vi "未命名 3.vi"() -> ()   [LabVIEW 2010]
uses:
  <vilib>/addons/Modulation/Analog/controls/Complex Data Waveform.ctl
  <vilib>/addons/Modulation/Digital/General/MT Generate Bits (Galois, PN Order).vi
  <vilib>/addons/Modulation/Digital/Impairments/Fading Profiles/MT Rician Fading Profile (Jakes).vi
  <vilib>/Analysis/2dsp.llb/Complex FFT.vi
  <vilib>/imath/engines/lvmath2/RunTimeEngine/ErrorHandling/NIMS_Finalize Error.vi
  <vilib>/imath/engines/lvmath2/RunTimeEngine/Managers/WorkSpace/UID Generator.vi
  <vilib>/imath/engines/lvmath2/RunTimeEngine/Managers/SymbolTable/Clear UID.vi
  <vilib>/imath/engines/lvmath2/RunTimeEngine/NodeEndStatement/NIMS_NodeEndStatement_Output.vi
  <instcachedir>/0/NIMS_NodeEndStatement_Output_53EC0D466D134D7ABD903AC30B43404B.lvgen/NIMS_NodeEndStatement_Output_53EC0D466D134D7ABD903AC30B43404B_000.vi
  <vilib>/imath/engines/lvmath2/RunTimeEngine/BuiltInFunctions/length/NIMS_length(GV).vi
  <instcachedir>/0/NIMS_length(GV)_08A3D13377FD4E4B96F5795FBF3698FA.lvgen/NIMS_length(GV)_08A3D13377FD4E4B96F5795FBF3698FA_002.vi
  <vilib>/imath/engines/lvmath2/RunTimeEngine/RunTimeType/NIMS_RunTimeType_From StrictType (excl LVString).vi
  <vilib>/imath/engines/lvmath2/RunTimeEngine/LocalVariableDefStatement/MC_LocalVariableDefStatement_Display.vi
  <vilib>/imath/engines/lvmath2/RunTimeEngine/BuiltInFunctions/zeros/NIMS_V=zeros(I32,I32).vi
  <vilib>/imathl/engines/lvmath/Functions/Error Handling/Create Error.vi
  <vilib>/imath/engines/lvmath2/RunTimeEngine/RangeToken/NIMS_Range_R2 - Integer.vi
  <instcachedir>/0/NIMS_Range_R2 - Integer_217CA55F27D14E80B3D190635C7B3F47.lvgen/NIMS_Range_R2 - Integer_217CA55F27D14E80B3D190635C7B3F47_000.vi
  <vilib>/imath/engines/lvmath2/RunTimeEngine/CommandStatement/MC_CommandStatement_break.vi
  <vilib>/imath/engines/lvmath2/RunTimeEngine/VariableToken/Read/NIMS_Get Elements - RV(_) - Check.vi
  <instcachedir>/0/NIMS_Get Elements - RV(_) - Check_1F6F8656162345078B1D4DC9877DFAE9.lvgen/NIMS_Get Elements - RV(_) - Check_1F6F8656162345078B1D4DC9877DFAE9_004.vi
  <vilib>/imath/engines/lvmath2/RunTimeEngine/ReplaceToken/NIMS_Replace - Check Linear.vi
  <instcachedir>/0/NIMS_Replace - Check Linear_662D5651E4E34E0584DA82A256193A4C.lvgen/NIMS_Replace - Check Linear_662D5651E4E34E0584DA82A256193A4C_002.vi
  <vilib>/imath/engines/lvmath2/RunTimeEngine/ReplaceToken/NIMS_Replace - Size Check _(_)=S.vi
  <instcachedir>/0/NIMS_Replace - Size Check _(_)=S_6CAC13ACC74349C582FDAB09BCDAB70F.lvgen/NIMS_Replace - Size Check _(_)=S_6CAC13ACC74349C582FDAB09BCDAB70F_001.vi
  <vilib>/imath/engines/lvmath2/RunTimeEngine/ReplaceToken/NIMS_Replace - V(S)=S.vi
  <instcachedir>/0/NIMS_Replace - V(S)=S_78FDB6CCD265407D8926E4CF958018EB.lvgen/NIMS_Replace - V(S)=S_78FDB6CCD265407D8926E4CF958018EB_001.vi
  <vilib>/Analysis/2dsp.llb/Inverse Complex FFT.vi
  <vilib>/addons/Modulation/niDMT.lvlib
  <vilib>/Analysis/NI_AALPro.lvlib
  <vilib>/addons/Modulation/niAMT.lvlib
  <vilib>/addons/Adaptive Filters/NI_AdaptiveFilter.lvlib
  <vilib>/addons/Modulation/Digital/Impairments/MT Apply Flat Fading Profile.vi
  <vilib>/imath/engines/lvmath2/RunTimeEngine/Managers/SymbolTable/NIMS_WorkSpace.lvlib
  <vilib>/addons/Adaptive Filters/Analysis/AFT Set Coefficients (FIR, Complex).vi
  <vilib>/addons/Adaptive Filters/Create/AFT Create FIR LMS (Complex).vi
  <vilib>/imath/engines/lvmath2/RunTimeEngine/BuiltInFunctions/zeros/NIMS_M=zeros(I32,I32).vi
  <vilib>/imath/engines/lvmath2/RunTimeEngine/ReplaceToken/NIMS_Replace - M(S,S)=S.vi
  <vilib>/imath/engines/lvmath2/RunTimeEngine/ReplaceToken/NIMS_Replace - Check Row.vi
  <vilib>/imath/engines/lvmath2/RunTimeEngine/ReplaceToken/NIMS_Replace - Check Column.vi
  <vilib>/imath/engines/lvmath2/RunTimeEngine/ReplaceToken/NIMS_Replace - Size Check M(_,_)=S.vi
  <vilib>/imath/engines/lvmath2/RunTimeEngine/ErrorHandling/NIMS_Create Error From Enums.vi
  <vilib>/addons/Adaptive Filters/Processing/AFT Filter Signal (Real, PtByPt).vi
  <vilib>/measure/NI_MABase.lvlib
panel:
  out "filter_out 5":dbl[](graph)
  out "coe":cdb[](array[numeric])
  out "filter_out 4":dbl[](graph)
  out "filter_out 3":dbl[](graph)
  out "filter_out 2":dbl[](graph)
  out "波形图 5":dbl[](graph)
  out "子数组":dbl[](graph)
  out "dout":cdb[][](array[numeric])
  out "波形图 4":dbl[](graph)
  out "波形图 3":dbl[](graph)
  out "波形图 2":dbl[](graph)
  out "波形图":dbl[](graph)
  out "constellation graph 2":T1(graph) caption="constellation graph"
  out "TX Constellation 2":T2(graph) caption="TX Constellation"
  out "Y":dbl[](graph)
  out "filter_out":dbl[](graph)
  out "TX Constellation":T2(graph)
  out "constellation graph":T1(graph)
  out "X":dbl[](graph)
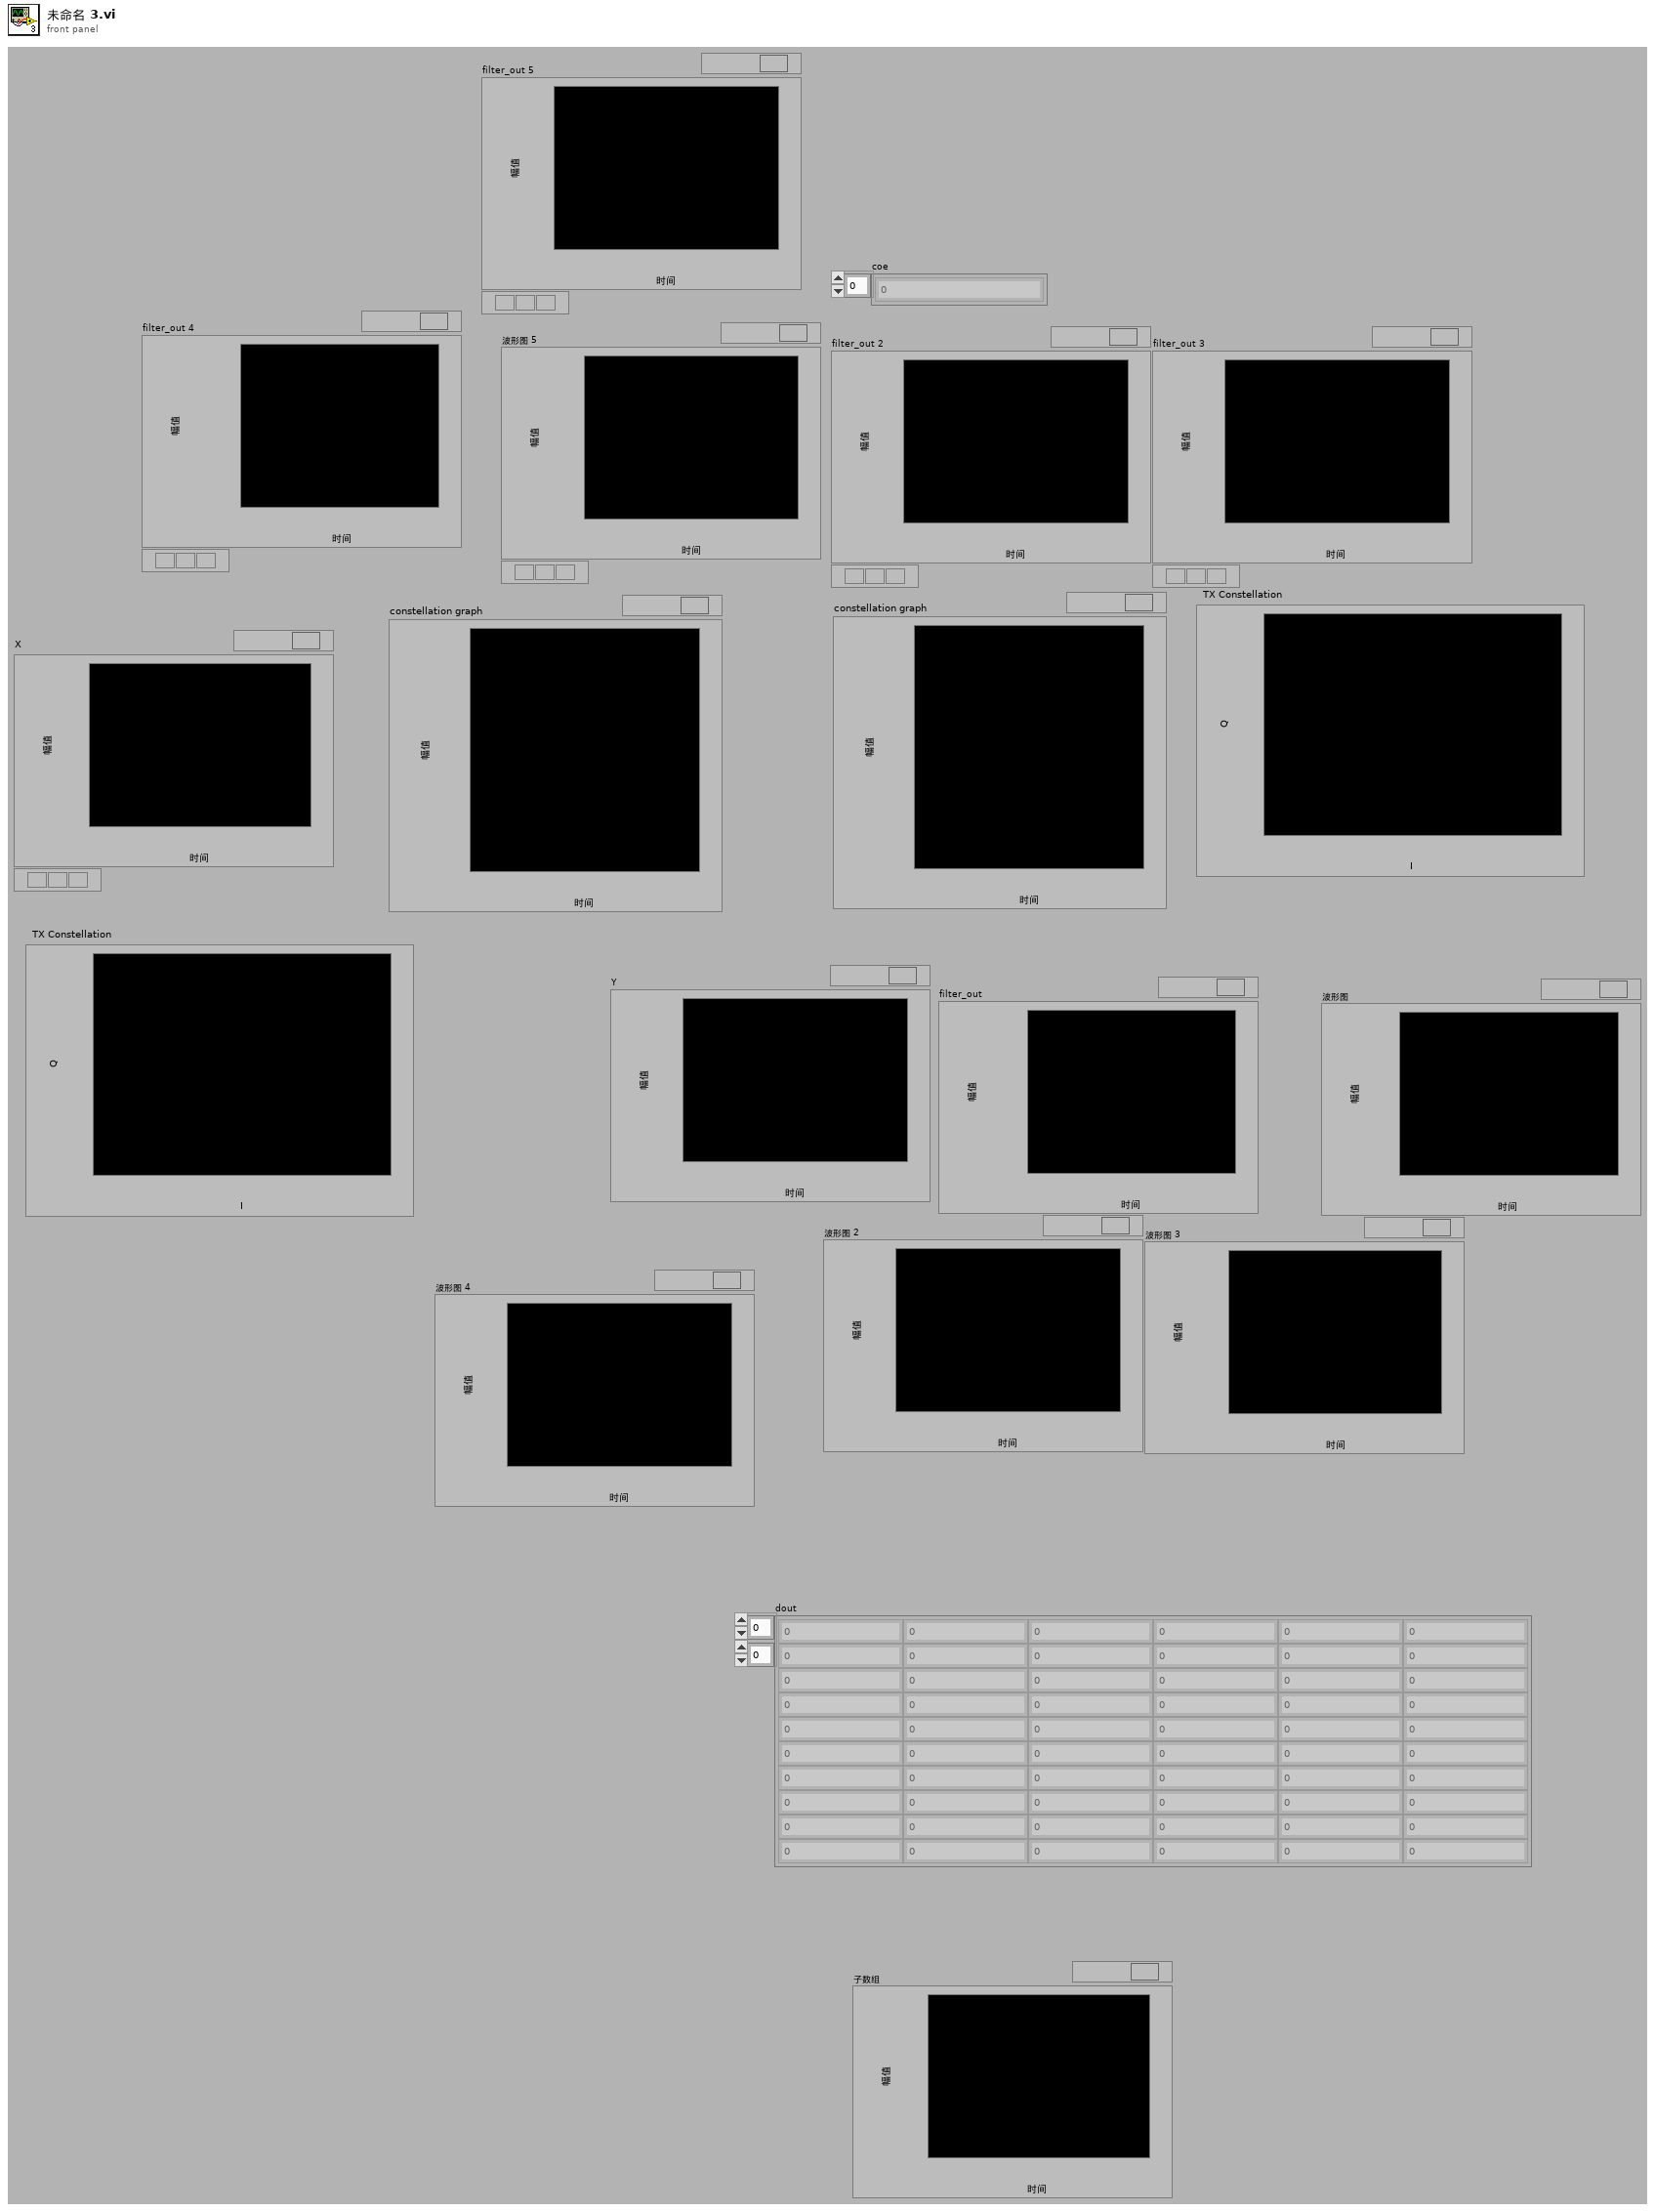
[diagram p1: front panel]
types:
  T1 = cluster{"constellation":dbl[], "oversampled data":dbl[]}[]
  T2 = cluster{"Decimated Array":dbl[], "Decimated Array":dbl[]}[]
  T3 = typedef "niAMT.lvlib/Complex Data Waveform.ctl" = cluster{"t0":dbl, "dt":dbl, "Y":cdb[]}
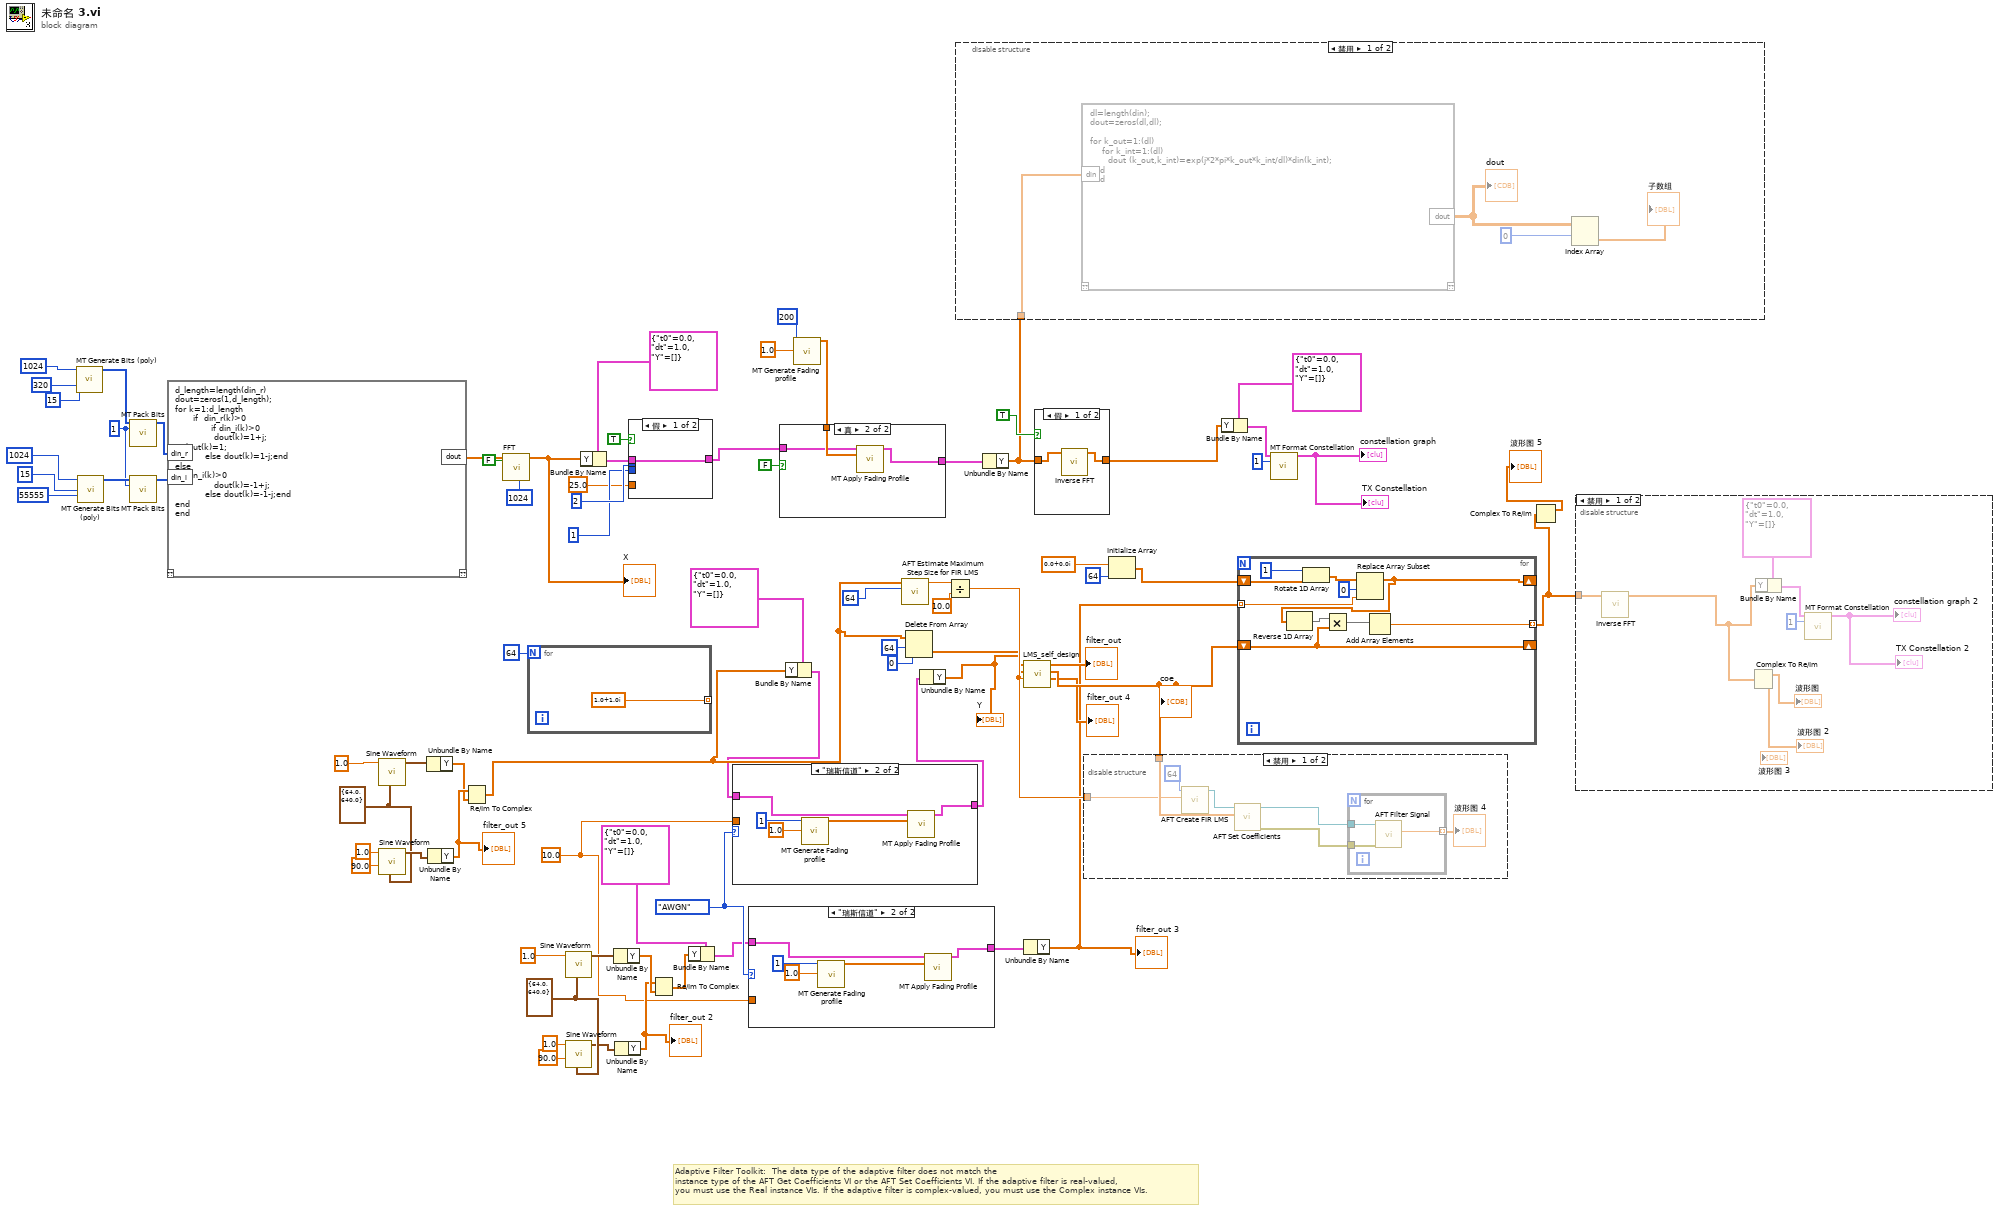
[diagram p0: block diagram]
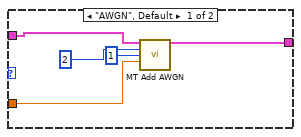
[diagram p3: hidden frame]
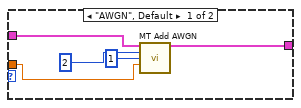
[diagram p6: hidden frame]
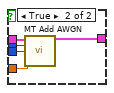
[diagram p8: hidden frame]
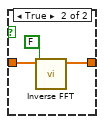
[diagram p9: hidden frame]
diagram:
  w4 = cluster{"Fs":dbl, "#s":dbl} {"Fs"=64.0, "#s"=640.0} ("sampling info")
  w23 = 10.0 ("Eb/N0 (10 dB)")
  w32 = cluster{"Fs":dbl, "#s":dbl} {"Fs"=64.0, "#s"=640.0} ("sampling info")
  w36 = enum16{"AWGN", "瑞斯信道"}."AWGN"
  w71 = 1 ("bits per integer")
  # "Adaptive Filter Toolkit:  The data type of the adaptive filter does not match the \ninstance type of the AFT Get Coefficients VI or the AFT Set Coefficients VI. If the adaptive filter is real-valued, \nyou must use the Real instance VIs. If the adaptive filter is complex-valued, you must use the Complex instance VIs."
  n1 = call-poly <vilib>:"MT Generate Bits (poly).vi"("total bits (128)"=1024, "PN sequence order (9)"=15, "seed in (0xD6BF7DF2)"=320) -> ("output bit stream"=w77:i8[])  [unwired: 10 in, 2 out]
  n2 = call-poly <vilib>:"MT Generate Bits (poly).vi"("total bits (128)"=1024, "PN sequence order (9)"=15, "seed in (0xD6BF7DF2)"=55555) -> ("output bit stream"=w73:i8[])  [unwired: 10 in, 2 out]
  n3 = call <vilib>:"MT Pack Bits.vi"("input bit stream"=w77, "bits per integer"=w71) -> ("output integers"=w68:i32[])  [unwired: 12 in, 1 out]
  n4 = call <vilib>:"MT Pack Bits.vi"("input bit stream"=w73, "bits per integer"=w71) -> ("output integers"=w69:i32[])  [unwired: 12 in, 1 out]
  n5 = mathscript code="d_length=length(din_r)\ndout=zeros(1,d_length);\nfor k=1:d_length\n      if  din_r(k)>0\n            if din_i(k)>0\n             dout(k)=1+j;\n%dout(k)=1;\n          else dout(k)=1-j;end\nelse   \n if din_i(k)>0\n             dout(k)=-1+j;\n          else dout(k)=-1-j;end\nend\nend"("din_r"=w68, "din_i"=w69) -> ("dout"=w56:cdb[])  [unwired: 1 in, 1 out]
  n6 = call <vilib>:"Sine Waveform.vi"("sampling info"=w4, "frequency"=1.0) -> ("signal out"=w8:waveform(dbl))  [unwired: 8 in, 1 out]
  n7 = call <vilib>:"Sine Waveform.vi"("sampling info"=w4, "phase"=90.0, "frequency"=1.0) -> ("signal out"=w9:waveform(dbl))  [unwired: 7 in, 1 out]
  n8 = Unbundle By Name(w8) -> ("Y"=w10:dbl[])
  n9 = Unbundle By Name(w9) -> ("Y"=w11:dbl[])
  "filter_out 5" <- w11
  n10 = Re/Im To Complex(1:w10, 2:w11) -> (0:w2:cdb[])
  n11 = call-poly <vilib>:"FFT.vi"("FFT size"=1024, "shift?"=FALSE, "X"=w56) -> ("FFT {X}"=w47:cdb[])  [unwired: 7 in, 1 out]
  "X" <- w47
  n12 = for {
    N: 64 -> [_]
    tunnel: [cdb 1.0+1.0i] -> _ mode=indexing
  }
  n13 = call <vilib>:"Sine Waveform.vi"("sampling info"=w32, "frequency"=1.0) -> ("signal out"=w31:waveform(dbl))  [unwired: 8 in, 1 out]
  n14 = call <vilib>:"Sine Waveform.vi"("sampling info"=w32, "phase"=90.0, "frequency"=1.0) -> ("signal out"=w30:waveform(dbl))  [unwired: 7 in, 1 out]
  n15 = Bundle By Name(cluster=T3 {"t0"=0.0, "dt"=1.0, "Y"=[]} ("input complex waveform"), "Y"=w47) -> (w65:T3)
  n16 = Unbundle By Name(w31) -> ("Y"=w29:dbl[])
  n17 = Unbundle By Name(w30) -> ("Y"=w25:dbl[])
  "filter_out 2" <- w25
  n18 = case shown="假" TRUE {
    tunnel: 2 ("samples per symbol (16)") -> [_ w85]
    tunnel: w65 -> [w80 w84]
    tunnel: 1 ("bits per symbol (1)") -> [_ w83]
    tunnel: 25.0 ("Eb/N0 (10 dB)") -> [_ w82]
    tunnel: [w80 w81] -> w51
    frame False {
    }
    frame True {
      n19 = call <vilib>:"MT Add AWGN.vi"("input complex waveform"=w84, "samples per symbol (16)"=w85, "bits per symbol (1)"=w83, "Eb/N0 (10 dB)"=w82) -> ("output complex waveform"=w81:T3)  [unwired: 9 in, 2 out]
    }
  }
  n20 = Re/Im To Complex(1:w29, 2:w25) -> (0:w15:cdb[])
  n21 = Bundle By Name(cluster=T3 {"t0"=0.0, "dt"=1.0, "Y"=[]} ("input complex waveform"), "Y"=w15) -> (w16:T3)
  n22 = case shown="\"瑞斯信道\"" w36 {
    tunnel: [w88 w92] -> w27
    tunnel: w16 -> [w87 w91]
    tunnel: w23 -> [w86 _]
    frame "AWGN", Default {
      n23 = call <vilib>:"MT Add AWGN.vi"("input complex waveform"=w87, "samples per symbol (16)"=2, "bits per symbol (1)"=1, "Eb/N0 (10 dB)"=w86) -> ("output complex waveform"=w88:T3)  [unwired: 9 in, 2 out]
    }
    frame "瑞斯信道" {
      n24 = call-poly <vilib>:"MT Generate Fading profile.vi"("profile length (samples)"=1, "sampling frequency (Hz)"=1.0) -> ("fading profile"=w95:cdb[])  [unwired: 11 in, 2 out]
      n25 = call-poly <vilib>:"MT Apply Fading Profile.vi"("input complex waveform"=w91, "fading profile"=w95) -> ("output complex waveform"=w92:T3)  [unwired: 12 in, 1 out]
    }
  }
  n26 = Bundle By Name(cluster=T3 {"t0"=0.0, "dt"=1.0, "Y"=[]} ("input complex waveform"), "Y"=w2) -> (w1:T3)
  n27 = case shown="\"瑞斯信道\"" w36 {
    tunnel: [w98 w101] -> w43
    tunnel: w1 -> [w97 w102]
    tunnel: w23 -> [w96 _]
    frame "AWGN", Default {
      n28 = call <vilib>:"MT Add AWGN.vi"("input complex waveform"=w97, "samples per symbol (16)"=2, "bits per symbol (1)"=1, "Eb/N0 (10 dB)"=w96) -> ("output complex waveform"=w98:T3)  [unwired: 9 in, 2 out]
    }
    frame "瑞斯信道" {
      n29 = call-poly <vilib>:"MT Generate Fading profile.vi"("profile length (samples)"=1, "sampling frequency (Hz)"=1.0) -> ("fading profile"=w105:cdb[])  [unwired: 11 in, 2 out]
      n30 = call-poly <vilib>:"MT Apply Fading Profile.vi"("input complex waveform"=w102, "fading profile"=w105) -> ("output complex waveform"=w101:T3)  [unwired: 12 in, 1 out]
    }
  }
  n31 = call-poly <vilib>:"MT Generate Fading profile.vi"("profile length (samples)"=200, "sampling frequency (Hz)"=1.0) -> ("fading profile"=w52:cdb[])  [unwired: 11 in, 2 out]
  n32 = case shown="真" FALSE {
    tunnel: w52 -> [_ w109]
    tunnel: w51 -> [w106 w108]
    tunnel: [w106 w107] -> w50
    frame False {
    }
    frame True {
      n33 = call-poly <vilib>:"MT Apply Fading Profile.vi"("input complex waveform"=w108, "fading profile"=w109) -> ("output complex waveform"=w107:T3)  [unwired: 12 in, 1 out]
    }
  }
  n34 = call <vilib>:"AFT Estimate Maximum Step Size for FIR LMS.vi"("filter length"=64, "x(n)"=w2) -> ("maximum step size"=w22:dbl)  [unwired: 8 in, 1 out]
  n35 = Delete From Array(array=w2, length=64 ("长度"), index=0 ("索引")) -> (deleted portion=w14:cdb[])  [unwired: 1 out]
  n36 = Unbundle By Name(w43) -> ("Y"=w13:cdb[])
  "Y" <- w13
  n37 = Divide(x=w22, y=10.0) -> (x/y=w17:dbl)
  n38 = Unbundle By Name(w50) -> ("Y"=w37:cdb[])
  n39 = disable-structure shown="禁用" {
    disable-tunnel: w37 -> [w110 _]
    frame Disabled {
      n40 = mathscript code="dl=length(din);\ndout=zeros(dl,dl);\n\nfor k_out=1:(dl)\n    for k_int=1:(dl)\n      dout (k_out,k_int)=exp(j*2*pi*k_out*k_int/dl)*din(k_int);\nend\nend"("din"=w110) -> ("dout"=w113:cdb[][])  [unwired: 1 in, 1 out]
      "dout" <- w113
      n41 = Index Array(array=w113, index (row)=0 ("索引 (行)")) -> (element=→"子数组":cdb[])  [unwired: 1 in]
    }
    frame Enabled {
    }
  }
  n42 = call "LMS_self_design.vi"("step_delta"=w17, "train"=w14, "sig"=w13) -> ("error"=→"filter_out 4":dbl[], "coe"=w42:cdb[], "filter_out"=→"filter_out":cdb[])  [unwired: 6 in]
  "coe" <- w42
  n43 = Unbundle By Name(w27) -> ("Y"=w3:cdb[])
  "filter_out 3" <- w3
  n44 = case shown="假" TRUE {
    tunnel: [w257 w259] -> w41
    tunnel: w37 -> [w256 w258]
    frame False {
      n45 = call-poly <vilib>:"Inverse FFT.vi"("FFT {X}"=w256) -> ("X"=w257:cdb[])  [unwired: 9 in, 1 out]
    }
    frame True {
      n46 = call-poly <vilib>:"Inverse FFT.vi"("shift?"=FALSE, "FFT {X}"=w258) -> ("X"=w259:cdb[])  [unwired: 8 in, 1 out]
    }
  }
  n47 = disable-structure shown="禁用" {
    disable-tunnel: w42 -> [w267 _]
    disable-tunnel: w17 -> [w261 _]
    frame Disabled {
      n48 = call-poly <vilib>:"AFT Create FIR LMS.vi"("step size"=w261, "filter length"=64) -> ("adaptive filter out"=w262:refnum<k20>)  [unwired: 8 in, 1 out]
      n49 = call-poly <vilib>:"AFT Set Coefficients.vi"("coefficients"=w267, "adaptive filter in"=w262) -> ("error out"=w265:errorcluster, "adaptive filter out"=w266:refnum<k20>)  [unwired: 8 in]
      n50 = for {
        tunnel: w266 -> [w270]
        tunnel: w265 -> [w269]
        tunnel: [w268] -> w264 mode=indexing
        n51 = call-poly <vilib>:"AFT Filter Signal.vi"("error in (no error)"=w269, "adaptive filter in"=w270) -> ("y(n)"=w268:dbl)  [unwired: 7 in, 2 out]
      }
      "波形图 4" <- w264
    }
    frame Enabled {
    }
  }
  n52 = Initialize Array(cdb 0.0+0.0i, 64 ("维数大小")) -> (w38:cdb[])
  n53 = Bundle By Name(cluster=T3 {"t0"=0.0, "dt"=1.0, "Y"=[]} ("waveform"), "Y"=w41) -> (w60:T3)
  n54 = for {
    tunnel: [w279] -> w26 mode=indexing
    shift-right: [w273] -> _
    shift-left: w38 -> [w277]
    tunnel: w3 -> [w274] mode=indexing
    shift-right: [w271] -> _
    shift-left: w42 -> [w271]
    n55 = Rotate 1D Array(1:w277, 2:1 ("n")) -> (0:w276:cdb[])
    n56 = Replace Array Subset(array=w276, new element=w274, index=0 ("索引")) -> (w273:cdb[])
    n57 = Reverse 1D Array(array=w273) -> (reversed array=w272:cdb[])
    n58 = Multiply(x=w272, y=w271) -> (x*y=w280:cdb[])
    n59 = Add Array Elements(numeric array=w280) -> (sum=w279:cdb)
  }
  n60 = call <vilib>:"MT Format Constellation.vi"("waveform"=w60, "samples per symbol"=1) -> ("constellation graph"=→"constellation graph" →"TX Constellation":T1)  [unwired: 12 in, 1 out]
  n61 = Complex To Re/Im(x + iy=w26) -> (x=→"波形图 5":dbl[])  [unwired: 1 out]
  n62 = disable-structure shown="禁用" {
    disable-tunnel: w26 -> [w282 _]
    frame Disabled {
      n63 = call-poly <vilib>:"Inverse FFT.vi"("FFT {X}"=w282) -> ("X"=w281:cdb[])  [unwired: 9 in, 1 out]
      n64 = Complex To Re/Im(x + iy=w281) -> (x=→"波形图":dbl[], y=→"波形图 2":dbl[])
      n65 = Bundle By Name(cluster=T3 {"t0"=0.0, "dt"=1.0, "Y"=[]} ("waveform"), "Y"=w281) -> (w286:T3)
      n66 = call <vilib>:"MT Format Constellation.vi"("waveform"=w286, "samples per symbol"=1) -> ("constellation graph"=→"constellation graph 2" →"TX Constellation 2":T1)  [unwired: 12 in, 1 out]
    }
    frame Enabled {
    }
  }
